vi "SA Camera Popup.vi"(9 "Port":u16=5801, 10 "New Image":T1, 11 "Remote Host":string="roborio-836-frc.local") -> ()   [LabVIEW 2015]
uses:
  <vilib>/vision/Image Controls.llb/IMAQ Image.ctl
panel:
  out "Right Camera":T1(plugin-control)
  out "Left Camera":T1(plugin-control)
  in  "stop":bool
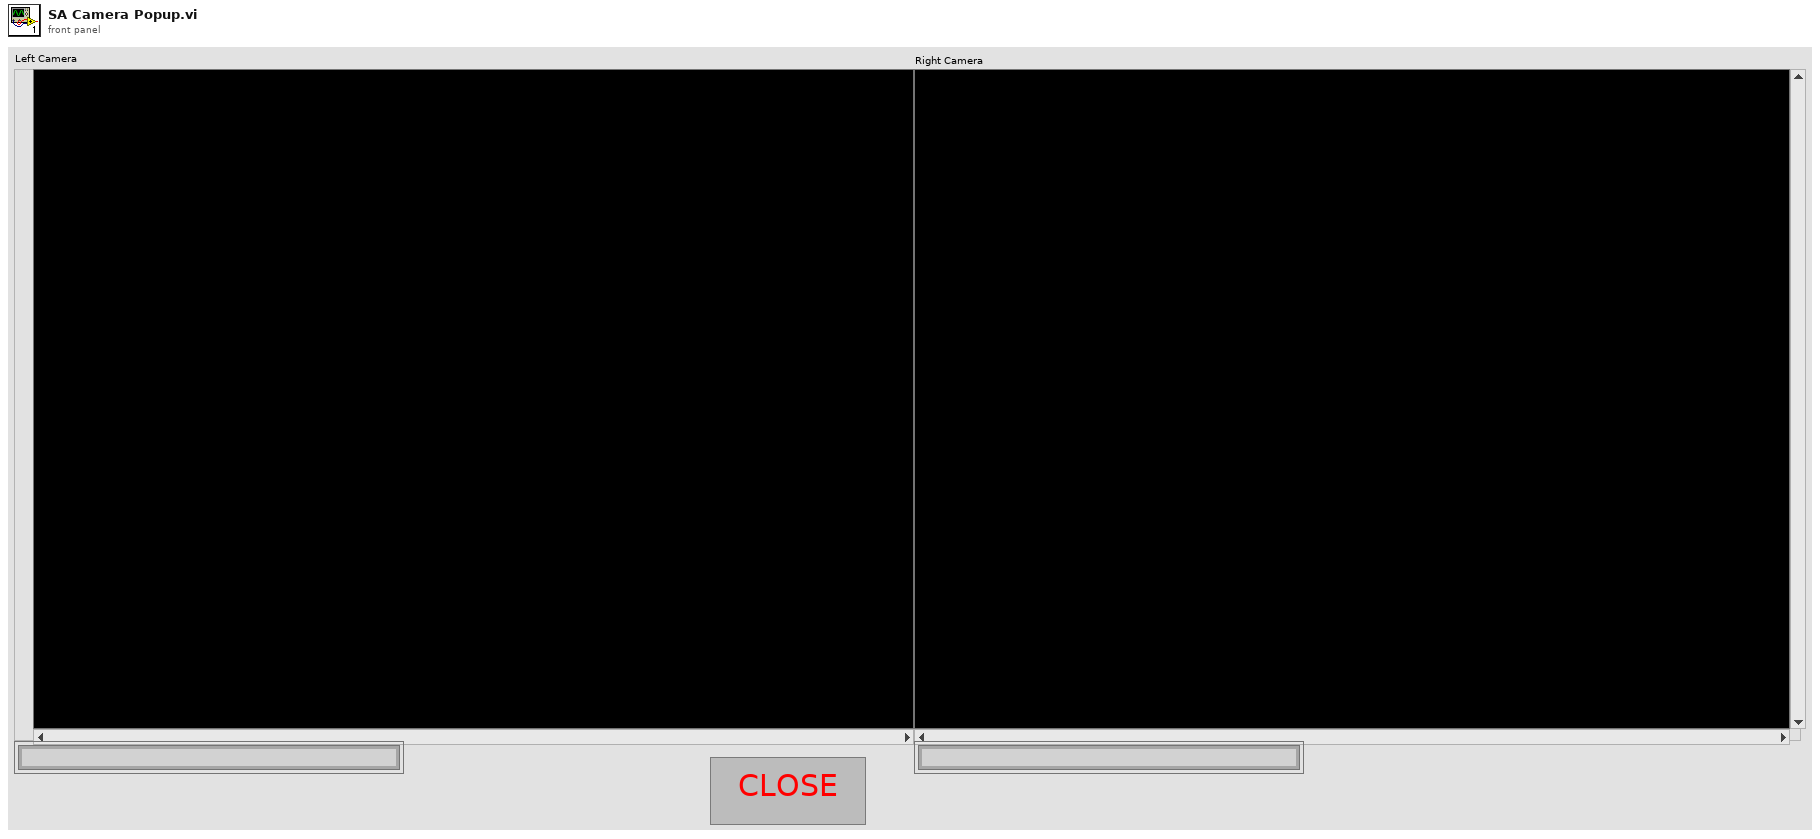
[diagram p1: front panel]
types:
  T1 = typedef "IMAQ Image.ctl" = refnum<image>
  T2 = typedef "Image Type" = u32
  T3 = typedef "Camera Network Settings.ctl" = cluster{"connection ID":refnum<k5>, "Port":u16, "Remote Host":string}
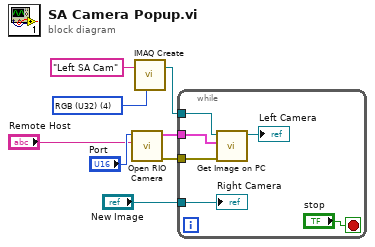
[diagram p0: block diagram]
diagram:
  w5 = T2 4 items=["Grayscale (U8)", "Grayscale (I16)", "Grayscale (SGL)", "Complex (CSG)", "RGB (U32)", "HSL (U32)", "RGB (U64)"] ("Image Type")
  n1 = call "Open RIO Camera.vi"("Remote Host"="Remote Host", "Port"="Port") -> ("error out"=w7:errorcluster, "Cluster"=w6:T3)  [unwired: 8 in]
  n2 = call "IMAQ Create"("Image Name"="Left SA Cam", "Image Type"=w5) -> ("New Image"=w3:T1)  [unwired: 2 in, 2 out]
  n3 = while {
    tunnel: w7 -> [w14]
    tunnel: w6 -> [w13]
    tunnel: w3 -> [w12]
    tunnel: "New Image" -> [w10]
    stop <- "stop" stop-if-true
    n4 = call "Get Image on PC.vi"("error in (no error)"=w14, "Cluster in"=w13, "Refnum in"=w12) -> ("Refnum out"=→"Left Camera":T1)  [unwired: 6 in, 2 out]
    "Right Camera" <- w10
  }
